vi "format display.vi"(9 "Display":enum16{"X and Y", "R and Theta"}(ring), 10 "Results (X,Y,R,Theta)":dbl[][](array[numeric]), 11 "t0":timestamp) -> (1 "Array 2":cluster{dbl[], dbl[]}[](array[cluster]), 2 "Array":waveform(dbl)[](array[waveform]), 3 "Array 3":waveform(dbl)[](array[waveform]))   [LabVIEW 2013]
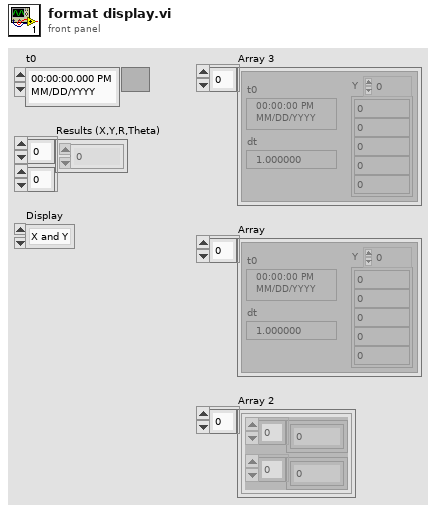
[diagram p1: front panel]
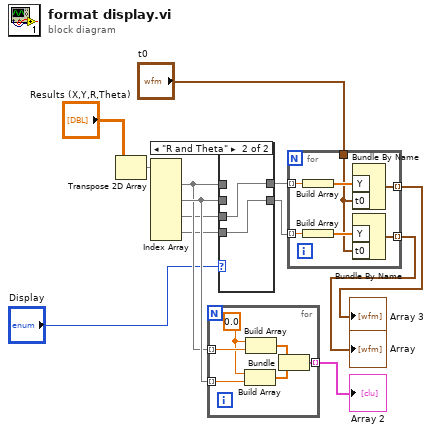
[diagram p0: block diagram]
diagram:
  n1 = Transpose 2D Array(2D array="Results (X,Y,R,Theta)") -> (transposed array=w1:dbl[][])
  n2 = Index Array(array=w1) -> (element #1=w10:dbl[], element #2=w11:dbl[], element #3=w4:dbl[], element #4=w5:dbl[])  [unwired: 8 in]
  n3 = for {
    tunnel: w10 -> [w19] mode=indexing
    tunnel: w11 -> [w18] mode=indexing
    tunnel: [w14] -> w12 mode=indexing
    w17 = 0.0
    n4 = Build Array(w17, w18) -> (w15:dbl[])
    n5 = Build Array(w17, w19) -> (w16:dbl[])
    n6 = Bundle(w16, w15) -> (w14:cluster{dbl[], dbl[]})  [unwired: 1 in]
  }
  "Array 2" <- w12
  n7 = case shown="\"R and Theta\"" "Display" {
    tunnel: w10 -> [w20 _]
    tunnel: [w20 w23] -> w6
    tunnel: w11 -> [w21 _]
    tunnel: [w21 w22] -> w7
    tunnel: w4 -> [_ w23]
    tunnel: w5 -> [_ w22]
    frame "X and Y", Default {
    }
    frame "R and Theta" {
    }
  }
  n8 = for {
    tunnel: w6 -> [w30] mode=indexing
    tunnel: w7 -> [w29] mode=indexing
    tunnel: [w28] -> w9 mode=indexing
    tunnel: [w27] -> w13 mode=indexing
    tunnel: "t0" -> [w24]
    n9 = Build Array(w30) -> (w26:dbl[])
    n10 = Build Array(w29) -> (w25:dbl[])
    n11 = Bundle By Name("Y"=w26, "t0"=w24) -> (w28:waveform(dbl))  [unwired: 1 in]
    n12 = Bundle By Name("Y"=w25, "t0"=w24) -> (w27:waveform(dbl))  [unwired: 1 in]
  }
  "Array" <- w13
  "Array 3" <- w9
